vi "Calibration Engine.vi"   [LabVIEW 2013]
types:
  T1 = cluster{"Calibrated":bool, "Load File":bool, "Error":errorcluster}
  T2 = enum16{"Engine Function", "Read Version", "Read Calibrated", "Read Load File", "Confirm File", "Read Confirmation"}
  T3 = enum16{"Engine Function", "Read Version", "Read Calibrated", "Read Load File", "Confirm File", "Read Confirmation", "Cal Engine Errors"}
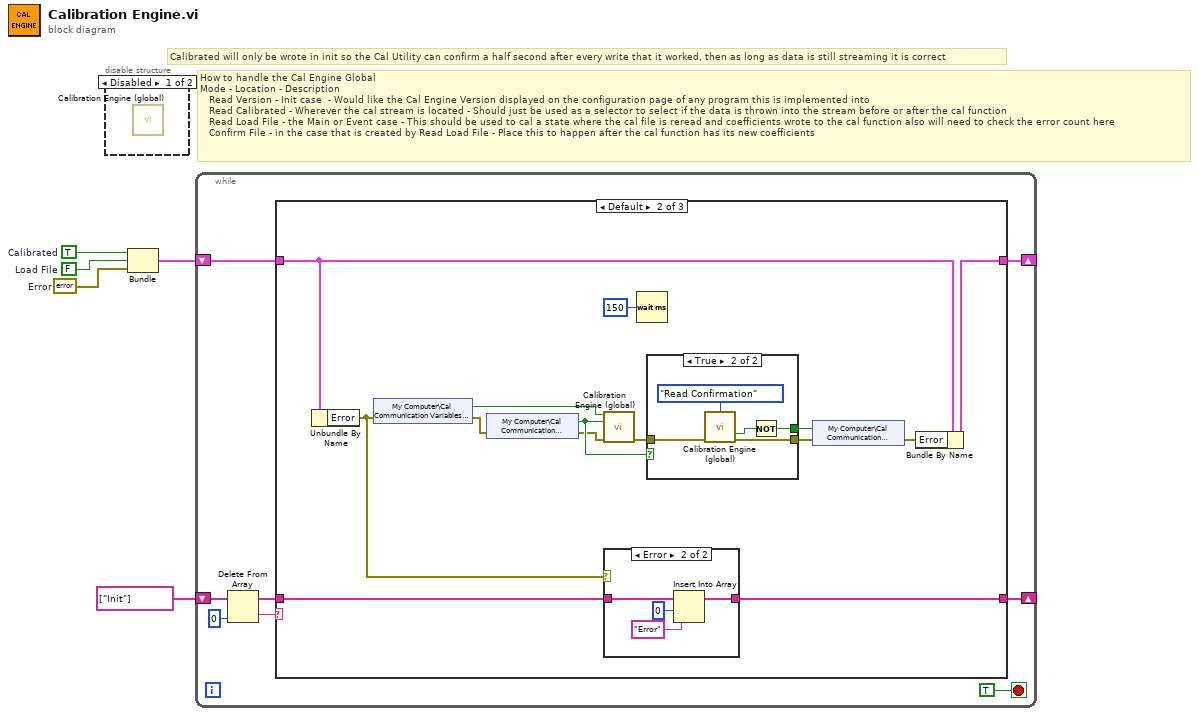
[diagram p0: block diagram]
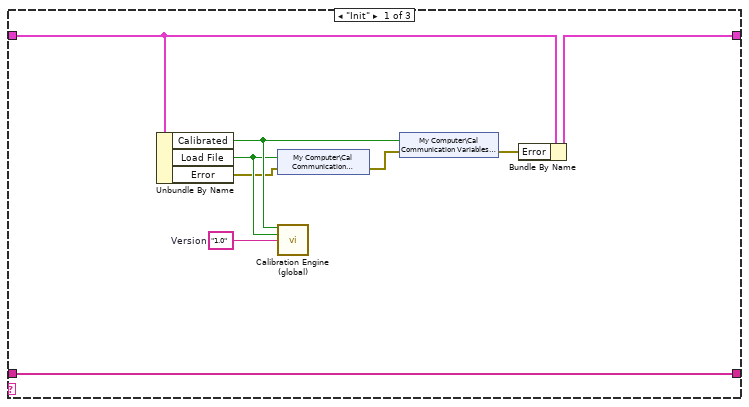
[diagram p3: hidden frame]
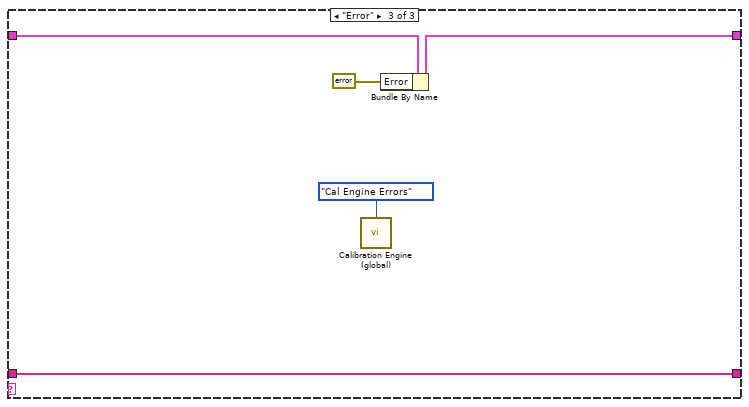
[diagram p6: hidden frame]
diagram:
  w1 = errorcluster {"status"=FALSE, "code"=0, "source"=""}  # Error
  w3 = FALSE  # Load File
  w4 = TRUE  # Calibrated
  # "How to handle the Cal Engine Global\nMode - Location - Description\n   Read Version - Init case  - Would like the Cal Engine Version displayed on the configuration page of any program this is implemented into\n   Read Calibrated - Wherever the cal stream is located - Should just be used as a selector to select if the data is thrown into the stream before or after the cal function\n   Read Load File - the Main or Event case - This should be used to cal a state where the cal file is reread and coefficients wrote to the cal function also will need to check the error count here\n   Confirm File - in the case that is created by Read Load File - Place this to happen after the cal function has its new coefficients"
  # "Calibrated will only be wrote in init so the Cal Utility can confirm a half second after every write that it worked, then as long as data is still streaming it is correct"
  n1 = disable-structure shown="Disabled" {
    frame Disabled {
      n2 = call "Calibration Engine (global).vi"() -> ()  [unwired: 10 in, 6 out]
    }
    frame Enabled {
    }
  }
  n3 = Bundle("Calibrated"=w4, "Load File"=w3, "Error"=w1) -> (w2:T1)  [unwired: 1 in]
  n4 = while {
    shift-right: [w8] -> _
    shift-left: string[] ["Init"] -> [w12]
    shift-right: [w6] -> _
    shift-left: w2 -> [w7]
    stop <- TRUE stop-if-true
    n5 = Delete From Array(array=w12, index=0) -> (deleted portion=w10:string, array with subset deleted=w9:string[])  [unwired: 1 in]
    n6 = case shown="Default" w10 {
      tunnel: w9 -> [w15 w30 w50]
      tunnel: [w15 w28 w50] -> w8
      tunnel: w7 -> [w21 w33 w52]
      tunnel: [w20 w32 w51] -> w6
      frame "Init" {
        w16 = "1.0"  # Version
        n7 = Unbundle By Name(w21) -> ("Calibrated"=w18:bool, "Load File"=w17:bool, "Error"=w14:errorcluster)
        n8 = shared-variable "My Computer\\Cal Communication Variables.lvlib\\Load File"(w17, error in=w14) -> (error out=w22:errorcluster)
        n9 = call "Calibration Engine (global).vi"("Calibrated In"=w18, "Load File In"=w17, "Version In"=w16) -> ()  [unwired: 7 in, 6 out]
        n10 = shared-variable "My Computer\\Cal Communication Variables.lvlib\\Calibrated"(w18, error in=w22) -> (error out=w19:errorcluster)
        n11 = Bundle By Name(cluster=w21, "Error"=w19) -> (w20:T1)
      }
      frame Default {
        n12 = Unbundle By Name(w33) -> ("Error"=w29:errorcluster)
        n13 = shared-variable "My Computer\\Cal Communication Variables.lvlib\\Calibrated"(error in=w29) -> (w35:bool, error out=w34:errorcluster)
        n14 = shared-variable "My Computer\\Cal Communication Variables.lvlib\\Load File"(error in=w34) -> (w27:bool, error out=w24:errorcluster)
        n15 = call "Calibration Engine (global).vi"("Calibrated In"=w35, "Load File In"=w27, "Error In"=w24) -> ("Error Out"=w25:errorcluster)  [unwired: 7 in, 5 out]
        n16 = case shown="Error" w29 {
          tunnel: w30 -> [w44 w48]
          tunnel: [w44 w47] -> w28
          frame No Error {
          }
          frame Error {
            n17 = Insert Into Array(array=w48, index=0, new element="Error" ("new element/subarray")) -> (w47:string[])
          }
        }
        n18 = Wait (ms)(milliseconds to wait=u32 150) -> ()  [unwired: 1 out]
        n19 = case shown="True" w27 {
          selector: w27 -> [w38 _]
          tunnel: [w38 w42] -> w26
          tunnel: w25 -> [w37 w41]
          tunnel: [w37 w40] -> w23
          frame False {
          }
          frame True {
            n20 = call "Calibration Engine (global).vi"("Mode"=T2."Read Confirmation", "Error In"=w41) -> ("File Loaded"=w39:bool, "Error Out"=w40:errorcluster)  [unwired: 8 in, 4 out]
            n21 = Not(x=w39) -> (.not. x?=w42:bool)
          }
        }
        n22 = shared-variable "My Computer\\Cal Communication Variables.lvlib\\Load File"(w26, error in=w23) -> (error out=w31:errorcluster)
        n23 = Bundle By Name(cluster=w33, "Error"=w31) -> (w32:T1)
      }
      frame "Error" {
        n24 = call "Calibration Engine (global).vi"("Mode"=T3."Cal Engine Errors") -> ()  [unwired: 9 in, 6 out]
        n25 = Bundle By Name(cluster=w52, "Error"=errorcluster {"status"=FALSE, "code"=0, "source"=""}) -> (w51:T1)
      }
    }
  }
